vi "PV ActiveLine - SensorIdentify.vi"(8 "Fehler (Eingang)":errorcluster, 11 "Referenz in":refnum<visa-resource-name>) -> (0 "Cluster (Ausgang)":errorcluster, 1 "Sensor 2":string, 2 "Sensor 1":string, 3 "Referenz out":refnum<visa-resource-name>)   [LabVIEW 2013, in "PV ActiveLine.lvlib"]
doc: "TID - Gauge Identification\n\nReceive: a,b\n\nIdentification gauge 1,\na =\nTPR/PCR (Pirani Gauge or Pirani Capacitance Gauge)\nIKR (Cold Cathode Gauge 10-9 and 10-11)\nPKR (FullRange® CC Gauge)\nPBR (FullRange® BA Gauge)\nIMR (Pirani / High Pressure Gauge)\nCMR/APR (Linear gauge\nnoSEn (no sensor)\nnoid (no identifier)\n\nIdentification gauge 2,\nb=\nTPR/PCR (Pirani Gauge or Pirani Capacitance Gauge)\nIKR (Cold Cathode Gauge 10-9 and 10-11)\nPKR (FullRange® CC Gauge)\nPBR (FullRange® BA Gauge)\nIMR (Pirani / High Pressure Gauge)\nCMR/APR (Linear gauge\nnoSEn (no sensor)\nnoid (no identifier)"
uses:
  C:/Program Files (x86)/National Instruments/LabVIEW 2013/PV ActiveLine/PV ActiveLine.lvlib
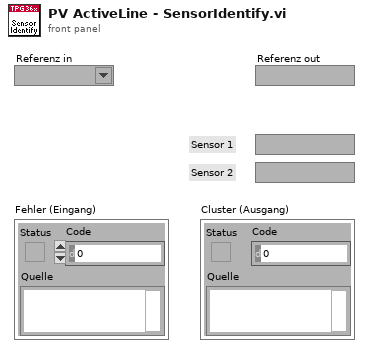
[diagram p1: front panel]
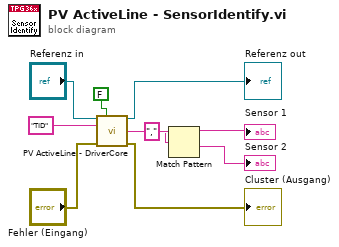
[diagram p0: block diagram]
diagram:
  n1 = call "PV ActiveLine - DriverCore.vi"("Referenz in"="Referenz in", "Write/Read"=FALSE, "Command"="TID", "Fehler (Eingang)"="Fehler (Eingang)") -> ("Referenz out"=→"Referenz out":refnum<visa-resource-name>, "String Out"=w8:string, "Cluster (Ausgang)"=→"Cluster (Ausgang)":errorcluster)  [unwired: 9 in]
  n2 = Match Pattern(string=w8, regular expression="," ("search char (-)")) -> (before substring=→"Sensor 1":string, after substring=→"Sensor 2":string)  [unwired: 1 in, 2 out]
